vi "Check The File Extension.vi"(8 "Error In":errorcluster, 10 "Expected File Extension (e.g \"txt\")":string, 11 "Filepath":path) -> (0 "Error Out":errorcluster)   [LabVIEW 2023, in "Error Manager.lvlib"]
uses:
  Error Manager.lvlib
panel:
  # "Input\nInputs to the VI"
  # "Development\nControls or indicators that are useful for development or testing, but which are not outputs of the VI."
  # "Output\nOutputs of the VI"
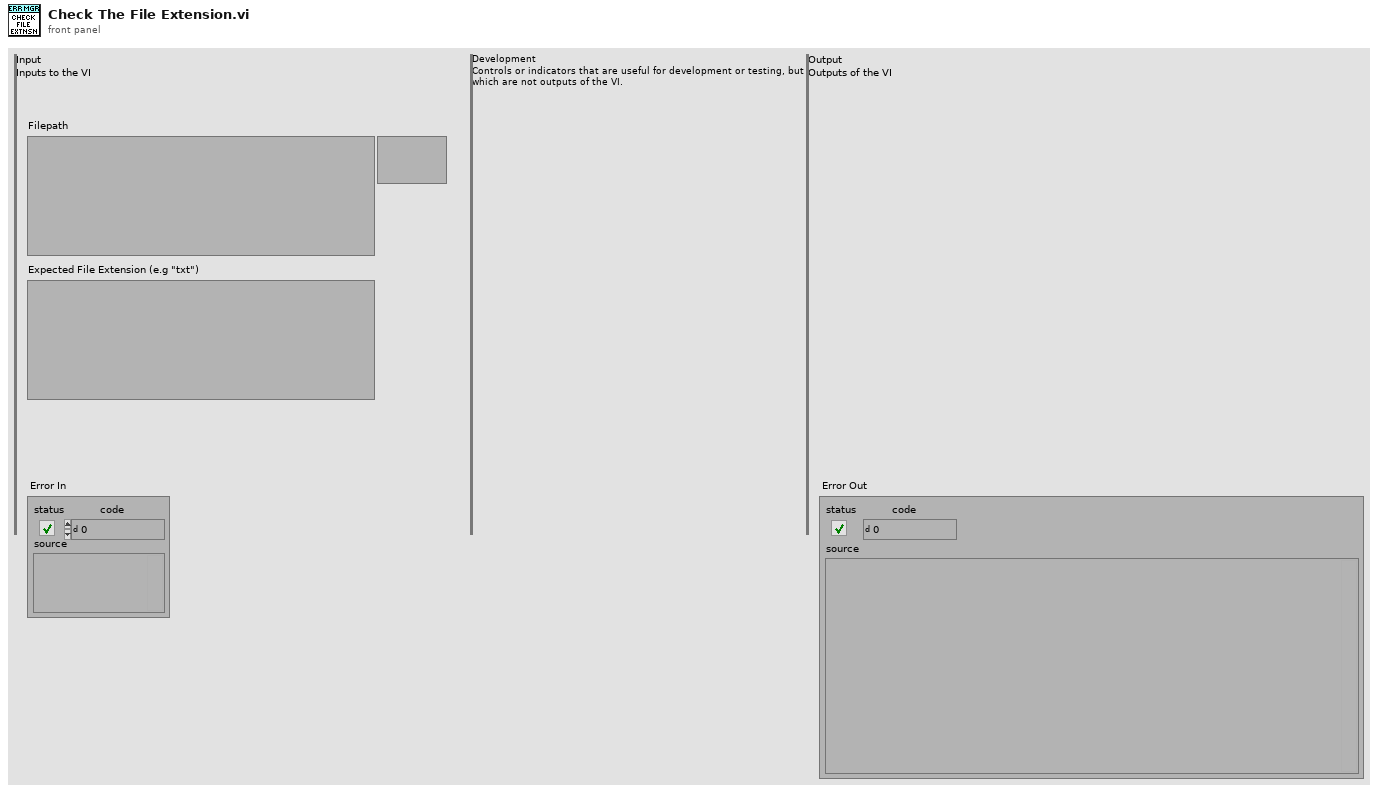
[diagram p1: front panel]
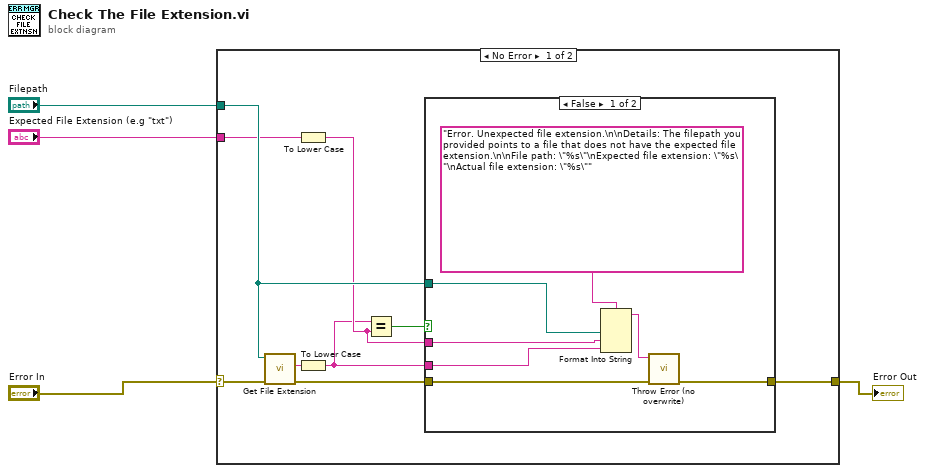
[diagram p0: block diagram]
diagram:
  n1 = case shown="No Error" "Error In" {
    selector: "Error In" -> [w13 w22]
    tunnel: "Filepath" -> [w9 _]
    tunnel: [w11 w22] -> w2
    tunnel: "Expected File Extension (e.g \"txt\")" -> [w8 _]
    frame No Error {
      n2 = call <vilib>:"Get File Extension.vi"("error in (no error)"=w13, "file"=w9) -> ("error out"=w12:errorcluster, "lowercase file extension"=w7:string)  [unwired: 5 in, 3 out]
      n3 = To Lower Case(string=w8) -> (all lower case string=w6:string)
      n4 = To Lower Case(string=w7) -> (all lower case string=w5:string)
      n5 = Equal?(x=w5, y=w6) -> (x = y?=w10:bool)
      n6 = case shown="False" w10 {
        tunnel: w12 -> [w20 w21]
        tunnel: [w19 w21] -> w11
        tunnel: w9 -> [w16 _]
        tunnel: w6 -> [w15 _]
        tunnel: w5 -> [w14 _]
        frame False {
          n7 = Format Into String(format string="Error. Unexpected file extension.\n\nDetails: The filepath you provided points to a file that does not have the expected file extension.\n\nFile path: \"%s\"\nExpected file extension: \"%s\"\nActual file extension: \"%s\"", w16, w15, w14) -> (resulting string=w17:string)  [unwired: 2 in, 1 out]
          n8 = call "Throw Error (no overwrite).vi"("error in"=w20, "Error Message (\"\")"=w17) -> ("error out"=w19:errorcluster)  [unwired: 9 in]
        }
        frame True {
        }
      }
    }
    frame Error {
    }
  }
  "Error Out" <- w2
